vi "Robot Global Data.vi"() -> ()   [LabVIEW 2020]
doc: "This global VI can contain as many global variables as you need. To create a global variable, place a control on the panel, give it a good name. To read or write to it from a VI, drag the icon to the diagram of that VI. You can also drag from the project. Click on the node to change which global you access. You shouldn't have multiple locations writing to a global or it will cause a race-condition."
uses:
  <vilib>/Rock Robotics/WPI/Camera/WPI_CameraImageSize.ctl
  <vilib>/Rock Robotics/WPI/DriverStation/WPI_DriverStationRobotMode2.ctl
panel:
  in  "Shooter Auto Setpoint":dbl=0.8 format="%#_13g"
  in  "Limelight Filepath":path
  in  "MaxDrive":dbl(slide)=0.6824817518248175 min=0.0 max=1.0 step=0.01 scale=0.0..1.0
  in  "DriveK":dbl(slide)=0.26277372262773724 min=0.0 max=1.0 step=0.05 scale=0.0..1.0
  in  "Limelight Goal Area":dbl(slide)=14.8723 min=0.1 max=25.0 step=0.25 scale=0.0..25.0
  in  "AimDeadband":dbl min=0.0 max=10.0 step=0.25
  in  "MinSteerCommand":dbl(slide)=0.2717391304347826 min=0.0 max=0.5 step=0.05 scale=0.0..0.5
  in  "SteeringK":dbl(slide)=0.025362318840579712 min=0.0 max=0.25 step=0.01 scale=0.0..0.25
  out "Drive with Limelight":bool
  in  "Shooter Setpoint Reverse":dbl=0.8 format="%#_13g"
  in  "Transfer Release Setpoint Reverse":dbl
  in  "Record Path Counter":dbl
  in  "Path Filename":path
  in  "Intake Reverse Setpoint":dbl=0.8 format="%#_13g"
  in  "Reverse Duration":dbl=3.0 format="%#_13g"
  in  "Intake Sped Up Setpoint":dbl=0.8 format="%#_13g"
  in  "Intake Sped Up Duration":dbl=3.0 format="%#_13g"
  in  "Custom MaxSpeedSlow (0.6)":dbl=0.6
  in  "Pivot Duration":dbl
  in  "Pivot Right Speed":dbl
  in  "Pivot Left Speed":dbl
  in  "Auto Pickup":string
  in  "Auto List":string
  in  "Spring Arm Setpoint":dbl
  in  "Climb Setpoint":dbl
  in  "Transfer Release Duration":dbl
  in  "Transfer Up Duration":dbl
  in  "Transfer Release Setpoint":dbl
  in  "Transfer Up Setpoint":dbl
  in  "Record Path":bool
  in  "Wheel":dbl
  in  "Throttle":dbl
  in  "Not Used Start":bool
  in  "Not Used Back":bool
  in  "Intake Reverse A":bool
  in  "Intake Sped Up B":bool
  in  "Not Used Right Stick Button":bool
  in  "Limelight Vision X":bool
  in  "Load Pipeline 1 Start":bool
  in  "Load Pipeline 0 Back":bool
  in  "Stop Limelight Right Stick Button":bool
  in  "Start Limelight Left Stick Button":bool
  in  "LED OFF B":bool
  in  "LED ON Y":bool
  in  "Limelight Camera A":bool
  in  "Record Path Stop RB":bool
  in  "Record Path Start LB":bool
  in  "Pivot Right RT":bool
  in  "Pivot Left LT":bool
  in  "Not Used Left Stick Button":bool
  in  "Transfer Release X":bool
  in  "Not Used Y":bool
  in  "Intake Arm Down LT":bool
  in  "Intake Arm Up LB":bool
  in  "Intake RT":bool
  in  "Shooter RB":bool
  in  "Intake Setpoint":dbl=0.8 format="%#_13g"
  in  "Intake Duration (s)":dbl=3.0 format="%#_13g"
  in  "Shooter Duration":dbl=3.0 format="%#_13g"
  in  "Shooter Setpoint":dbl=0.8 format="%#_13g"
  in  "Robot Mode":T1
  in  "image size":T2=enum."320x240"
  in  "Enable Vision":bool
  # "DRIVER"
  # "OPERATOR"
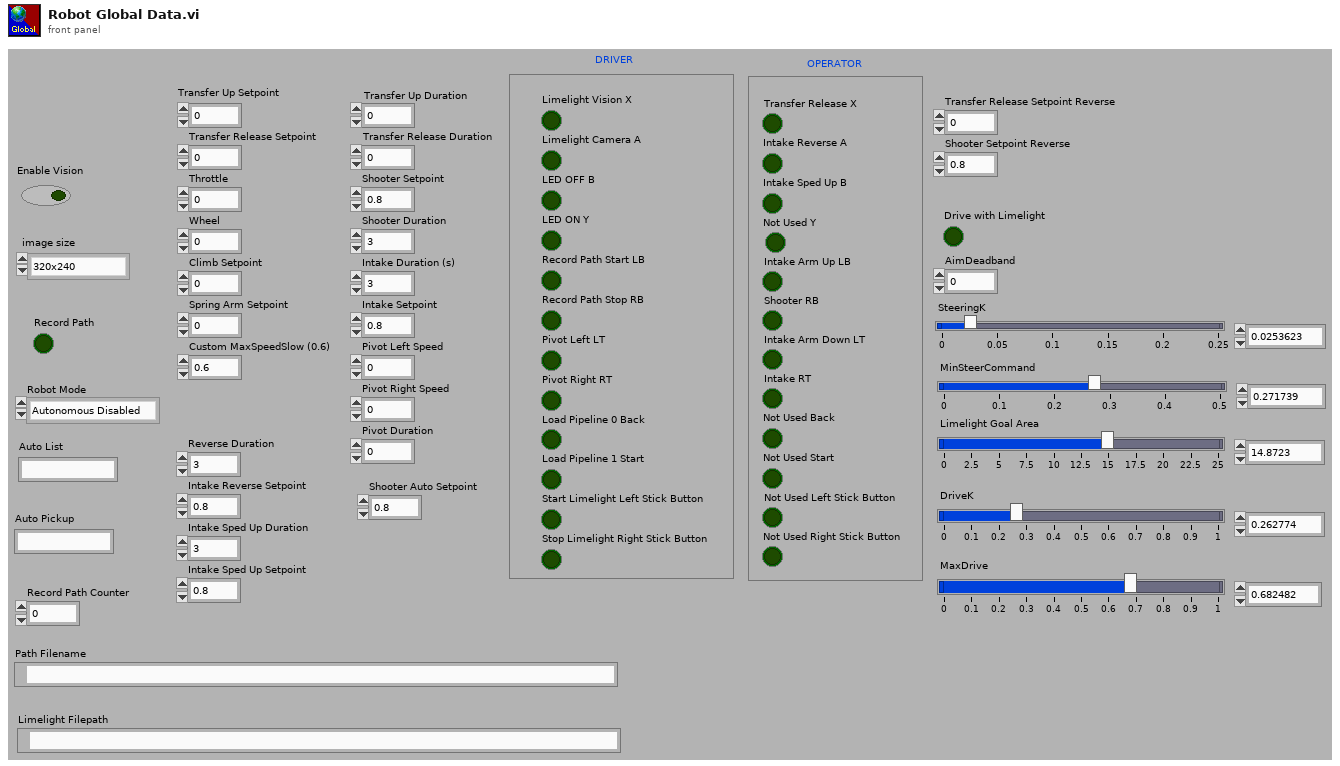
[diagram p1: front panel]
types:
  T1 = typedef "WPI_DriverStationRobotMode2.ctl" = enum16{"Autonomous Disabled", "Autonomous Enabled", "Teleop Disabled", "Teleop Enabled", "Disconnected", "Finish", "Test Disabled", "Test Enabled", "Emergency Stopped"}
  T2 = typedef "WPI_CameraImageSize.ctl" = enum16{"640x480", "320x240", "160x120", "Custom"}
diagram:
